vi "WPI_SerialPortRead.vi"(8 "error in (no error)":errorcluster, 10 "Num Bytes to Read":u32, 11 "SerialPortRef":T1) -> (0 "error out":errorcluster, 2 "Buffer":string, 3 "SerialPortRef":T1)   [LabVIEW 2017]
doc: "Reads a specified number of bytes from the serial device you specify.\n\nThis software is licensed. Open the labview\\readme\\WPI Robotics Library Open Source License.txt file for more information."
uses:
  <vilib>/Rock Robotics/WPI/SerialPort/WPI_SerialPortRef.ctl
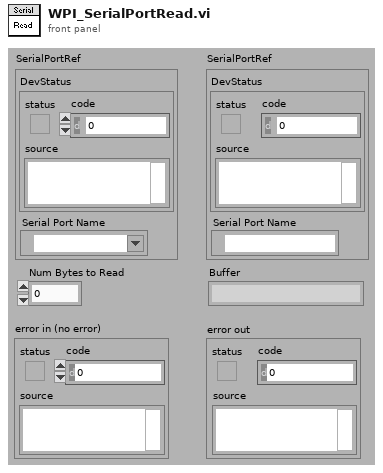
[diagram p1: front panel]
types:
  T1 = typedef "WPI_SerialPortRef.ctl" = cluster{"DevStatus":errorcluster, "Serial Port Name":refnum<visa-resource-name>}
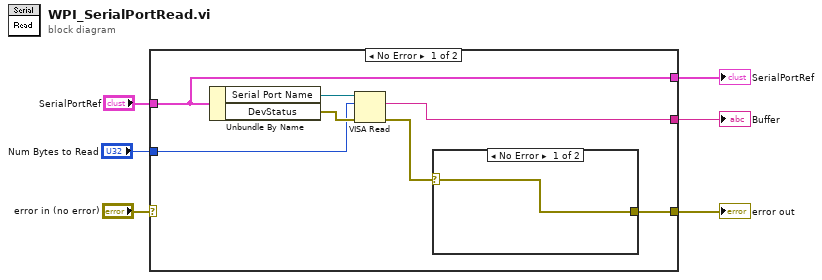
[diagram p0: block diagram]
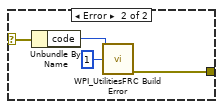
[diagram p2: hidden frame]
diagram:
  n1 = case shown="No Error" "error in (no error)" {
    selector: "error in (no error)" -> [_ w20]
    tunnel: "SerialPortRef" -> [w7 w19]
    tunnel: [w7 w19] -> w5
    tunnel: [w8 w20] -> w3
    tunnel: [w10 _] -> w2
    tunnel: "Num Bytes to Read" -> [w11 _]
    frame No Error {
      n2 = Unbundle By Name(w7) -> ("Serial Port Name"=w13:refnum<visa-resource-name>, "DevStatus"=w12:errorcluster)
      n3 = VISA Read(VISA resource name=w13, byte count=w11, error in (no error)=w12) -> (read buffer=w10:string, error out=w9:errorcluster)  [unwired: 2 out]
      n4 = case shown="No Error" w9 {
        selector: w9 -> [w14 w16]
        tunnel: [w14 w15] -> w8
        frame No Error {
        }
        frame Error {
          n5 = Unbundle By Name(w16) -> ("code"=w18:i32)
          n6 = call <vilib>:"WPI_UtilitiesFRC Build Error.vi"("error code"=w18, "chain levels to remove (1)"=1) -> ("error out"=w15:errorcluster)  [unwired: 3 in, 10 out]
        }
      }
    }
    frame Error {
    }
  }
  "error out" <- w3
  "SerialPortRef" <- w5
  "Buffer" <- w2
